vi "Saturn JTAG Startup.vi"(11 "error in (no error)":errorcluster) -> (15 "error out":errorcluster)   [LabVIEW 2010]
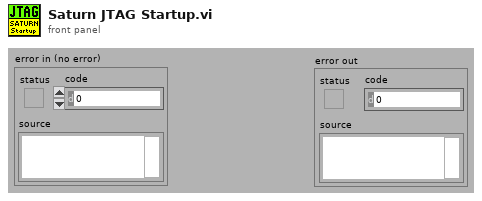
[diagram p1: front panel]
types:
  T1 = enum8{"PORT_OUT", "PORT_SEL", "PORT_RES_EN", "READ_PORT", "PORT_DIR", "SET_LCM", "PLUTO_WRITE_SINGLE", "PLUTO_READ_SINGLE", "PLUTO_WRITE_MASK", "STIM_POWER_UP", "STIM_POWER_DN", "SATURN_WRITE_SINGLE", "SATURN_READ_SINGLE", "SATURN_WRITE_BLOCK", "SATURN_READ_BLOCK", "SATURN_WRITE_MASK", "MICS_POWER_UP", "MICS_POWER_DN", "MICS_WRITE_SINGLE", "MICS_READ_SINGLE", "MICS_WRITE_BLOCK", "MICS_READ_BLOCK", "MICS_WRITE_MASK", "MEM_POWER_UP", "MEM_POWER_DN", "MEM_WRITE_SINGLE", "MEM_READ_SINGLE", "MEM_WRITE_BLOCK", "MEM_READ_BLOCK", "MEM_WRITE_MASK", "MEM_WRITE_SR", "MEM_READ_SR", "MEM_OPCODE", "INIT_VARIABLES", "DCO -> 1 MHz", "DCO -> 8 MHz", "START_STIM_CLK", "STOP_STIM_CLK", "PULSE_STIM_CLK", "PULSE_STIM_SCK", "SINGLE_ADC12", "SINGLE_ADC12_REPEAT", "MULTI_ADC12", "MULTI_ADC12_REPEAT", "Disable_ADC12", "READ_IO_VARIABLES"}
  T2 = enum16{"PWR LDOA_EN BIT", "PWR VD1_EN BIT", "PWR VD2_EN BIT", "PWR VD3_EN BIT", "PWR VD4_EN BIT", "PWR BFG_EN BIT", "PWR TEMP_EN BIT", "PWR THERM_EN BIT", "PWR CHARGE_EN BIT", "PWR COMP_OV BIT", "PWR MSPBUF < MSPBUF_IN", "PWR MSPBUF < Fuel Gauge", "PWR MSPBUF < Recharge PM", "PWR MSPBUF < Temp_Out", "PWR MSPBUF < Therm_Bias", "PWR MSPBUF < Therm_Input", "PWR MSPBUF < Therm_Offset", "PWR MSPBUF OFF", "PWR ASK_POL BIT", "PWR MAGSW_DISABLE BIT", "PWR MAGTIME_SEL 00 (OFF)", "PWR MAGTIME_SEL 01 (5S)", "PWR MAGTIME_SEL 10 (2S)", "PWR MAGTIME_SEL 11 (TEST)", "PWR STROBE_INT_EN BIT", "PWR STROBE_PW SET", "PWR STROBE_FREQ SET", "PWR HCM_PW SET", "PWR LCM_DC SET"}
  T3 = enum16{"Read Port Value", "Set Port Value", "Set Port Direction", "Set Port Select", "Set Port Res En"}
  T4 = enum16{"Manual Inputs", "PWR_LDO_EN", "PWR_STROBE_IN", "PWR_UV_PROT", "PWR_MAG_TO_OVRD", "PWR_BBC_CTL", "PWR_HVDD_CONN", "<Reserved_1>", "<Reserved_2>", "STIM_RUN", "STIM_STOP", "STIM_CONT", "STIM_SEL", "RST_N", "<Reserved_3>", "TETS_TXD", "<Reserved_4>", "<Reserved_5>", "PWR_MAG_SW (IN)", "PWR_MAG_2S (IN)", "PWR_MAG_5S (IN)", "TETS_RXD (IN)", "PWR_V_DET (IN)", "PWR_BRWN_OUT (IN)", "MICS_IRQ", "<Reserved_7>", "STIM_PROG (IN)", "STIM_PAUSE (IN)", "STIM_SYNC (IN)", "STIM_TFLG (IN)", "STIM_ERR (IN)"}
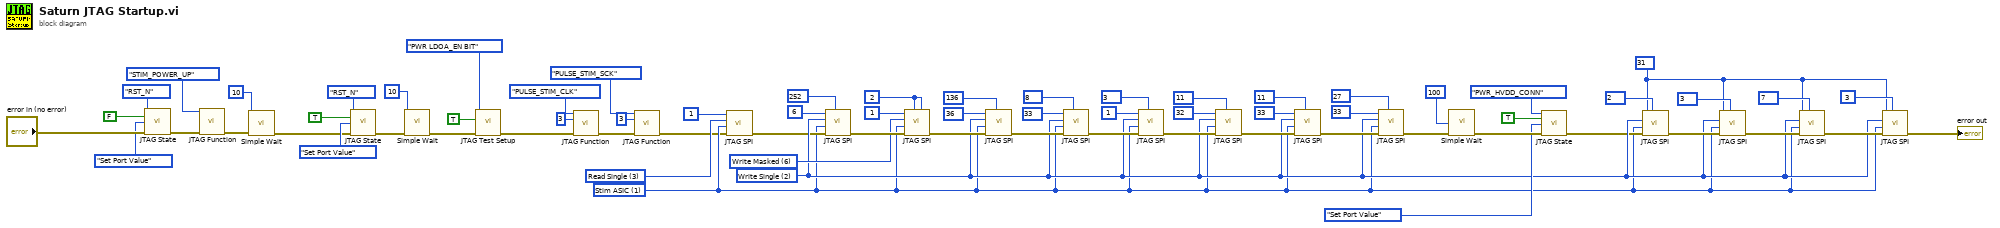
[diagram p0: block diagram]
diagram:
  w21 = u16 3 items=["Power UP", "Power DN", "Write Single", "Read Single", "Write Block", "Read Block", "Write Masked", "Test Value"] ("Function")
  w30 = u16 31 ("Address")
  w65 = u16 6 items=["Power UP", "Power DN", "Write Single", "Read Single", "Write Block", "Read Block", "Write Masked", "Test Value"] ("Function")
  w32 = u16 2 items=["Power UP", "Power DN", "Write Single", "Read Single", "Write Block", "Read Block", "Write Masked", "Test Value"] ("Function")
  w20 = u16 1 items=["Power ASIC", "Stim ASIC", "MICS Radio", "FRAM"] ("Target")
  w64 = u8 2 ("Single Write/Test")
  n1 = call "JTAG State.vi"("Quick Bit Function (Manual)"=T4."RST_N", "State (L)"=FALSE, "Function"=T3."Set Port Value", "error in (no error)"="error in (no error)") -> ("error out"=w26:errorcluster)  [unwired: 9 in, 2 out]
  n2 = call "JTAG Function.vi"("Enum"=T1."STIM_POWER_UP", "error in (no error)"=w26) -> ("error out"=w10:errorcluster)  [unwired: 11 in, 2 out]
  n3 = call "Simple Wait.vi"("mS"=u32 10, "error in"=w10) -> ("error out"=w11:errorcluster)  [unwired: 12 in, 1 out]
  n4 = call "JTAG State.vi"("Quick Bit Function (Manual)"=T4."RST_N", "State (L)"=TRUE, "Function"=T3."Set Port Value", "error in (no error)"=w11) -> ("error out"=w8:errorcluster)  [unwired: 9 in, 2 out]
  n5 = call "Simple Wait.vi"("mS"=u32 10, "error in"=w8) -> ("error out"=w7:errorcluster)  [unwired: 12 in, 1 out]
  n6 = call "JTAG Test Setup.vi"("error in (no error)"=w7, "BIT Value"=TRUE, "Test Function"=T2."PWR LDOA_EN BIT") -> ("error out"=w6:errorcluster)  [unwired: 8 in]
  n7 = call "JTAG Function.vi"("Enum"=T1."PULSE_STIM_CLK", "ARG 1"=u16 3, "error in (no error)"=w6) -> ("error out"=w16:errorcluster)  [unwired: 10 in, 2 out]
  n8 = call "JTAG Function.vi"("Enum"=T1."PULSE_STIM_SCK", "ARG 1"=u16 3, "error in (no error)"=w16) -> ("error out"=w15:errorcluster)  [unwired: 10 in, 2 out]
  n9 = call "JTAG SPI.vi"("error in (no error)"=w15, "Target"=w20, "Function"=w21, "Address"=u16 1) -> ("error out"=w22:errorcluster)  [unwired: 4 in, 3 out]
  n10 = call "JTAG SPI.vi"("Value"=u8 252 ("Single Write/Test"), "error in (no error)"=w22, "Target"=w20, "Function"=w32, "Address"=u16 6) -> ("error out"=w67:errorcluster)  [unwired: 3 in, 3 out]
  n11 = call "JTAG SPI.vi"("Mask"=w64, "Value"=w64, "error in (no error)"=w67, "Target"=w20, "Function"=w65, "Address"=u16 1) -> ("error out"=w63:errorcluster)  [unwired: 2 in, 3 out]
  n12 = call "JTAG SPI.vi"("Value"=u8 136 ("Single Write/Test"), "error in (no error)"=w63, "Target"=w20, "Function"=w32, "Address"=u16 36) -> ("error out"=w60:errorcluster)  [unwired: 3 in, 3 out]
  n13 = call "JTAG SPI.vi"("Value"=u8 8 ("Single Write/Test"), "error in (no error)"=w60, "Target"=w20, "Function"=w32, "Address"=u16 33) -> ("error out"=w57:errorcluster)  [unwired: 3 in, 3 out]
  n14 = call "JTAG SPI.vi"("Value"=u8 3 ("Single Write/Test"), "error in (no error)"=w57, "Target"=w20, "Function"=w32, "Address"=u16 1) -> ("error out"=w54:errorcluster)  [unwired: 3 in, 3 out]
  n15 = call "JTAG SPI.vi"("Value"=u8 11 ("Single Write/Test"), "error in (no error)"=w54, "Target"=w20, "Function"=w32, "Address"=u16 32) -> ("error out"=w51:errorcluster)  [unwired: 3 in, 3 out]
  n16 = call "JTAG SPI.vi"("Value"=u8 11 ("Single Write/Test"), "error in (no error)"=w51, "Target"=w20, "Function"=w32, "Address"=u16 33) -> ("error out"=w48:errorcluster)  [unwired: 3 in, 3 out]
  n17 = call "JTAG SPI.vi"("Value"=u8 27 ("Single Write/Test"), "error in (no error)"=w48, "Target"=w20, "Function"=w32, "Address"=u16 33) -> ("error out"=w44:errorcluster)  [unwired: 3 in, 3 out]
  n18 = call "Simple Wait.vi"("mS"=u32 100 ("milliseconds to wait"), "error in"=w44) -> ("error out"=w43:errorcluster)  [unwired: 12 in, 1 out]
  n19 = call "JTAG State.vi"("Quick Bit Function (Manual)"=T4."PWR_HVDD_CONN", "State (L)"=TRUE, "Function"=T3."Set Port Value", "error in (no error)"=w43) -> ("error out"=w23:errorcluster)  [unwired: 9 in, 2 out]
  n20 = call "JTAG SPI.vi"("Value"=u8 2 ("Single Write/Test"), "error in (no error)"=w23, "Target"=w20, "Function"=w32, "Address"=w30) -> ("error out"=w38:errorcluster)  [unwired: 3 in, 3 out]
  n21 = call "JTAG SPI.vi"("Value"=u8 3 ("Single Write/Test"), "error in (no error)"=w38, "Target"=w20, "Function"=w32, "Address"=w30) -> ("error out"=w36:errorcluster)  [unwired: 3 in, 3 out]
  n22 = call "JTAG SPI.vi"("Value"=u8 7 ("Single Write/Test"), "error in (no error)"=w36, "Target"=w20, "Function"=w32, "Address"=w30) -> ("error out"=w34:errorcluster)  [unwired: 3 in, 3 out]
  n23 = call "JTAG SPI.vi"("Value"=u8 3 ("Single Write/Test"), "error in (no error)"=w34, "Target"=w20, "Function"=w32, "Address"=w30) -> ("error out"=→"error out":errorcluster)  [unwired: 3 in, 3 out]
